vi "GetAllSpecialPixelInformation.vi"(8 "error in (no error)":errorcluster, 9 "block":u32, 10 "sample":u32, 11 "camera_pos":u16) -> (0 "error out":errorcluster, 3 "Cluster":T1)   [LabVIEW 2015, in "ESLSCDLL.lvlib"]
uses:
  ESLSCDLL.lvlib
  Globals.vi
panel:
  out "cameraSystem3030":bool
  out "cameraSystem3010":bool
  out "cameraSystem3001":bool
  out "impactSignal2":u32
  out "impactSignal1":u32
  out "s2State":bool
  out "s1State":bool
  out "scanIndex2":u32
  out "scanIndex":u32
  out "blockIndex":u32
  out "tempGood":bool
  out "overTemp":bool
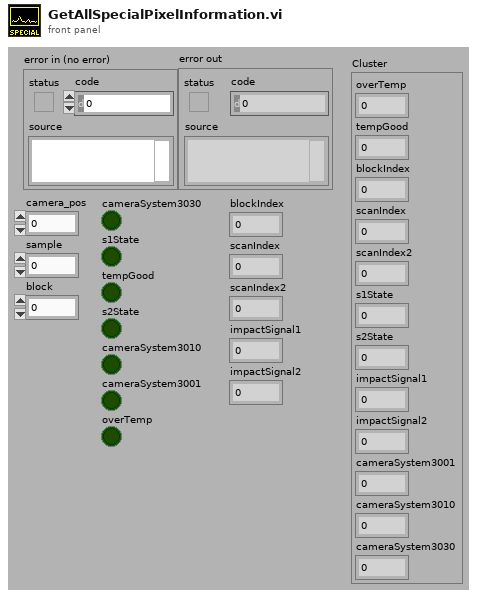
[diagram p1: front panel]
types:
  T1 = cluster{"overTemp":u32, "tempGood":u32, "blockIndex":u32, "scanIndex":u32, "scanIndex2":u32, "s1State":u32, "s2State":u32, "impactSignal1":u32, "impactSignal2":u32, "cameraSystem3001":u32, "cameraSystem3010":u32, "cameraSystem3030":u32}
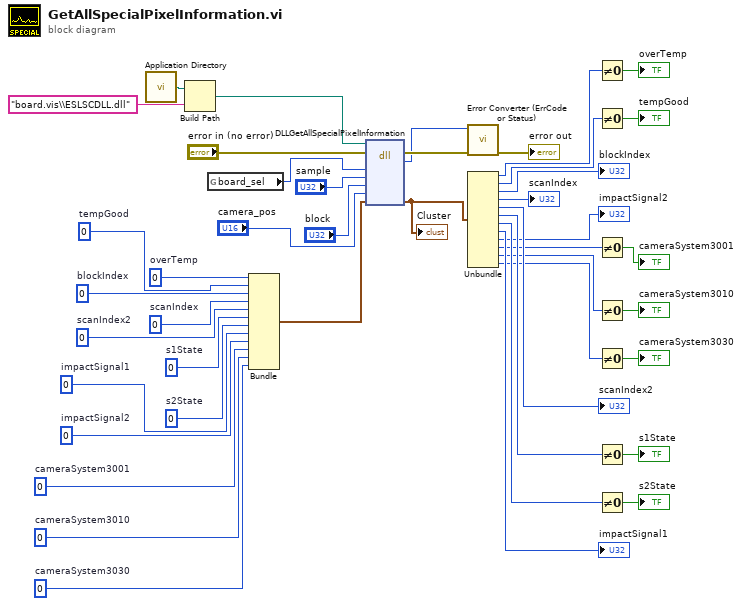
[diagram p0: block diagram]
diagram:
  w21 = u32 0  # cameraSystem3030
  w22 = u32 0  # cameraSystem3010
  w23 = u32 0  # cameraSystem3001
  w24 = u32 0  # impactSignal2
  w25 = u32 0  # impactSignal1
  w26 = u32 0  # s2State
  w27 = u32 0  # s1State
  w28 = u32 0  # scanIndex2
  w29 = u32 0  # scanIndex
  w30 = u32 0  # blockIndex
  w31 = u32 0  # tempGood
  w32 = u32 0  # overTemp
  n1 = call <vilib>:"Application Directory.vi"() -> ("Application Directory"=w40:path)
  n2 = Build Path(base path=w40, name or relative path="board.vis\\ESLSCDLL.dll") -> (appended path=w38:path)
  n3 = global read "Globals.vi" "board_sel"() -> (w37:u32)
  n4 = Bundle("overTemp"=w32, "tempGood"=w31, "blockIndex"=w30, "scanIndex"=w29, "scanIndex2"=w28, "s1State"=w27, "s2State"=w26, "impactSignal1"=w25, "impactSignal2"=w24, "cameraSystem3001"=w23, "cameraSystem3010"=w22, "cameraSystem3030"=w21) -> (w33:T1)  [unwired: 1 in]
  n5 = dll-call lib="C:/ENTW/PCIE/LV64/board.vis/ESLSCDLL.dll" fn="DLLGetAllSpecialPixelInformation" ("lwlscdll.dll:DLLWriteLongS0")(path in=w38, error in="error in (no error)", "board_sel"=w37, "sample"="sample", "block"="block", "camera_pos"="camera_pos", "special_pixels"=w33) -> (error out=w42:errorcluster, "es_status_codes"=w41:i32, "special_pixels"=w20:T1)  [unwired: 5 in, 1 out]
  "Cluster" <- w20
  n6 = call "Error Converter (ErrCode or Status).vi"("error in (no error)"=w42, "error code"=w41) -> ("error out"=→"error out":errorcluster)  [unwired: 9 in]
  n7 = Unbundle(w20) -> ("overTemp"=w19:u32, "tempGood"=w17:u32, "blockIndex"=→"blockIndex":u32, "scanIndex"=→"scanIndex":u32, "scanIndex2"=→"scanIndex2":u32, "s1State"=w12:u32, "s2State"=w10:u32, "impactSignal1"=→"impactSignal1":u32, "impactSignal2"=→"impactSignal2":u32, "cameraSystem3001"=w6:u32, "cameraSystem3010"=w5:u32, "cameraSystem3030"=w4:u32)
  n8 = Not Equal To 0?(x=w19) -> (x != 0?=→"overTemp":bool)
  n9 = Not Equal To 0?(x=w17) -> (x != 0?=→"tempGood":bool)
  n10 = Not Equal To 0?(x=w6) -> (x != 0?=→"cameraSystem3001":bool)
  n11 = Not Equal To 0?(x=w5) -> (x != 0?=→"cameraSystem3010":bool)
  n12 = Not Equal To 0?(x=w4) -> (x != 0?=→"cameraSystem3030":bool)
  n13 = Not Equal To 0?(x=w12) -> (x != 0?=→"s1State":bool)
  n14 = Not Equal To 0?(x=w10) -> (x != 0?=→"s2State":bool)
